vi "Encoder Input.vi"() -> ()   [LabVIEW 2009, in "MicroDAQ.lvlib"]
uses:
  <instrlib>/MicroDAQ/MicroDAQ.lvlib
  <instrlib>/MicroDAQ/Tools/Encoder type.ctl
  <instrlib>/MicroDAQ/Channel/Encoder/Create.vi
  <instrlib>/MicroDAQ/Channel/Encoder/Encoder.lvclass
panel:
  in  "Channel":T1=1 items=["ENC1"=1, "ENC2"=2]
  out "Position":i32
  out "Direction":enum16{"None", "CW", "CCW"}(ring)
  in  "IP address":string="10.10.1.1"
  in  "Stop":bool
  # "Device settings"
  # "Channel Settings"
  # "Read Values"
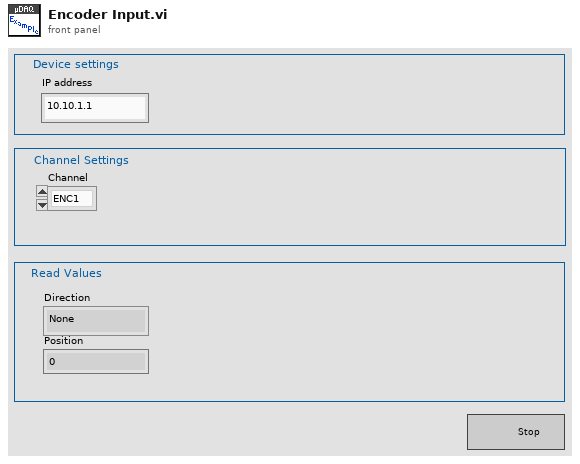
[diagram p1: front panel]
types:
  T1 = typedef "MicroDAQ.lvlib/Encoder type.ctl" = u8
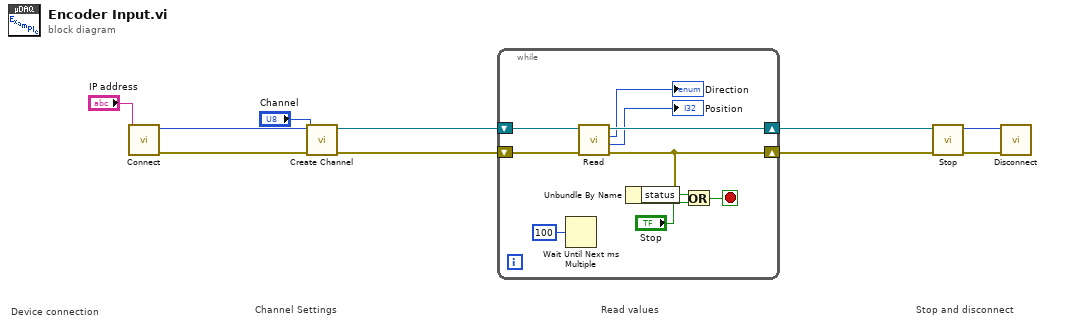
[diagram p0: block diagram]
diagram:
  # "Device connection"
  # "Read values"
  # "Stop and disconnect"
  # "Channel Settings"
  n1 = call <instrlib>:"Connect.vi"("IP address"="IP address") -> ("error out"=w7:errorcluster, "connection ID"=w8:i32)  [unwired: 9 in]
  n2 = call-poly <instrlib>:"Create Channel.vi"("error in (no error)"=w7, "Channel"="Channel", "connection ID"=w8) -> ("error out"=w9:errorcluster, "Task out"=w10:refnum<class "Encoder.lvclass">)  [unwired: 7 in]
  n3 = while {
    shift-right: [w15] -> w5
    shift-left: w10 -> [w17]
    shift-right: [w14] -> w4
    shift-left: w9 -> [w16]
    stop <- w18 stop-if-true
    n4 = Wait Until Next ms Multiple(millisecond multiple=u32 100) -> ()  [unwired: 1 out]
    n5 = call-poly <instrlib>:"Read.vi"("error in (no error)"=w16, "MicroDAQ.lvlib:Encoder.lvclass"=w17) -> ("error out"=w14:errorcluster, "position"=→"Position":i32, "direction"=→"Direction":enum16{"None", "CW", "CCW"}, "MicroDAQ.lvlib:Encoder.lvclass out"=w15:refnum<class "Encoder.lvclass">)  [unwired: 6 in]
    n6 = Unbundle By Name(w14) -> ("status"=w11:bool)
    n7 = Or(x=w11, y="Stop") -> (x .or. y?=w18:bool)
  }
  n8 = call-dynamic "Stop.vi"("error in (no error)"=w4, "Task in"=w5) -> ("error out"=w2:errorcluster, "connection ID"=w3:i32)  [unwired: 8 in]
  n9 = call <instrlib>:"Disconnect.vi"("error in (no error)"=w2, "connection ID"=w3) -> ()  [unwired: 9 in, 1 out]
